vi "G2131-i仪器串口通讯.vi"(0 "VISA resource name":refnum<visa-resource-name>="COM3", 2 "baud rate (9600)":u32=9600) -> (1 "Delta2Min":string, 5 "H2O":string, 6 "12CO2":string, 7 "12CO2(dry）":string, 8 "Delta5Min":string, 9 "13CO2":string, 10 "13CO2（dry）":string)   [LabVIEW 2016]
uses:
  <vilib>/Instr/_visa.llb/VISA Configure Serial Port (Instr).vi
panel:
  out "返回数 2":u32
  out "read buffer":string
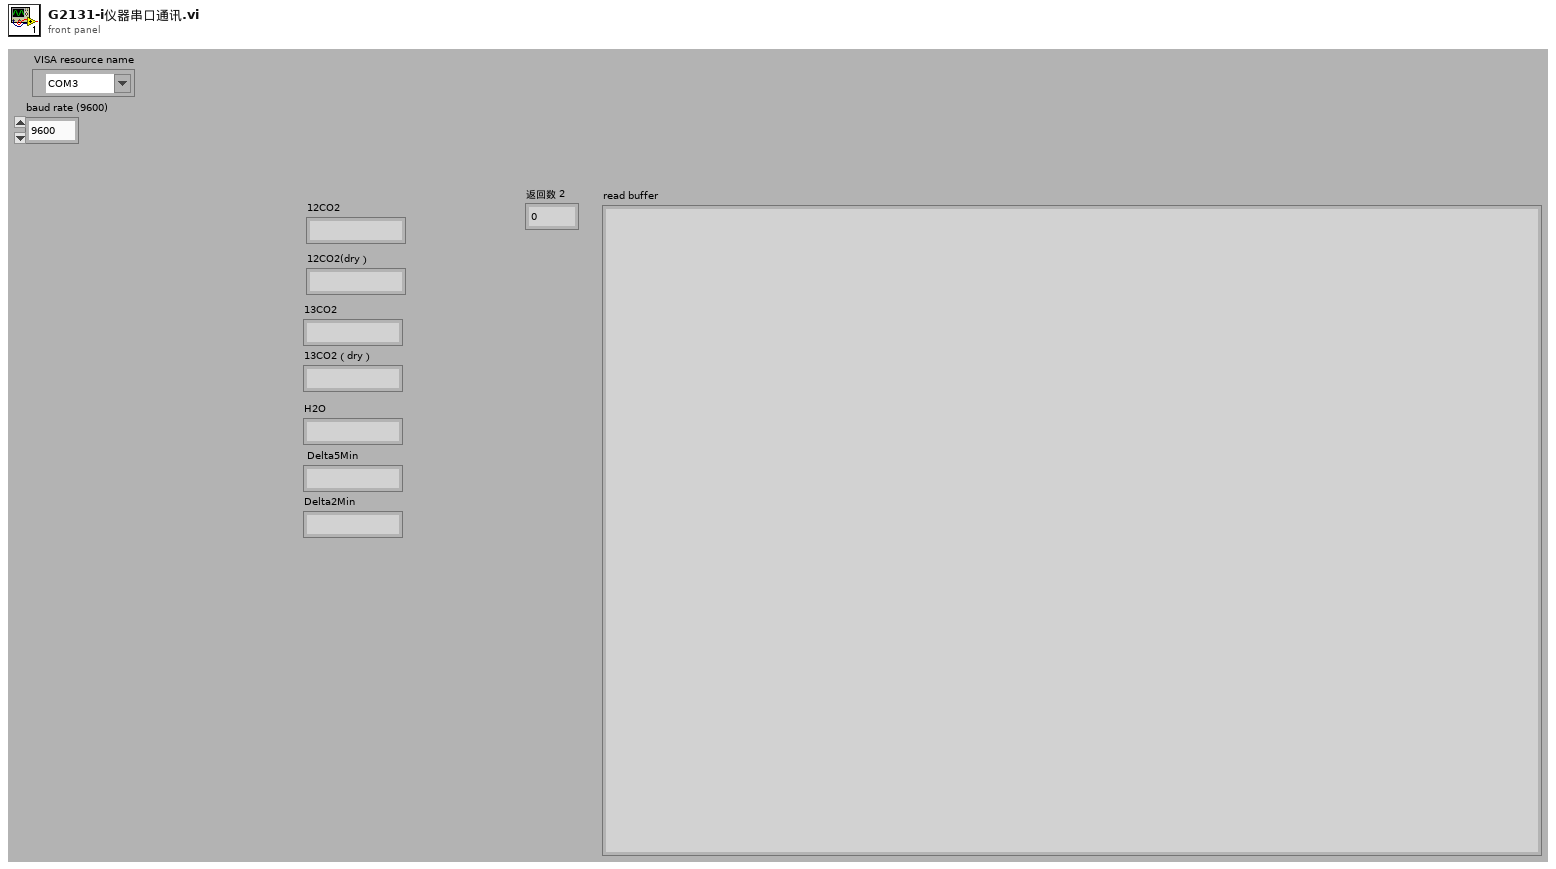
[diagram p1: front panel]
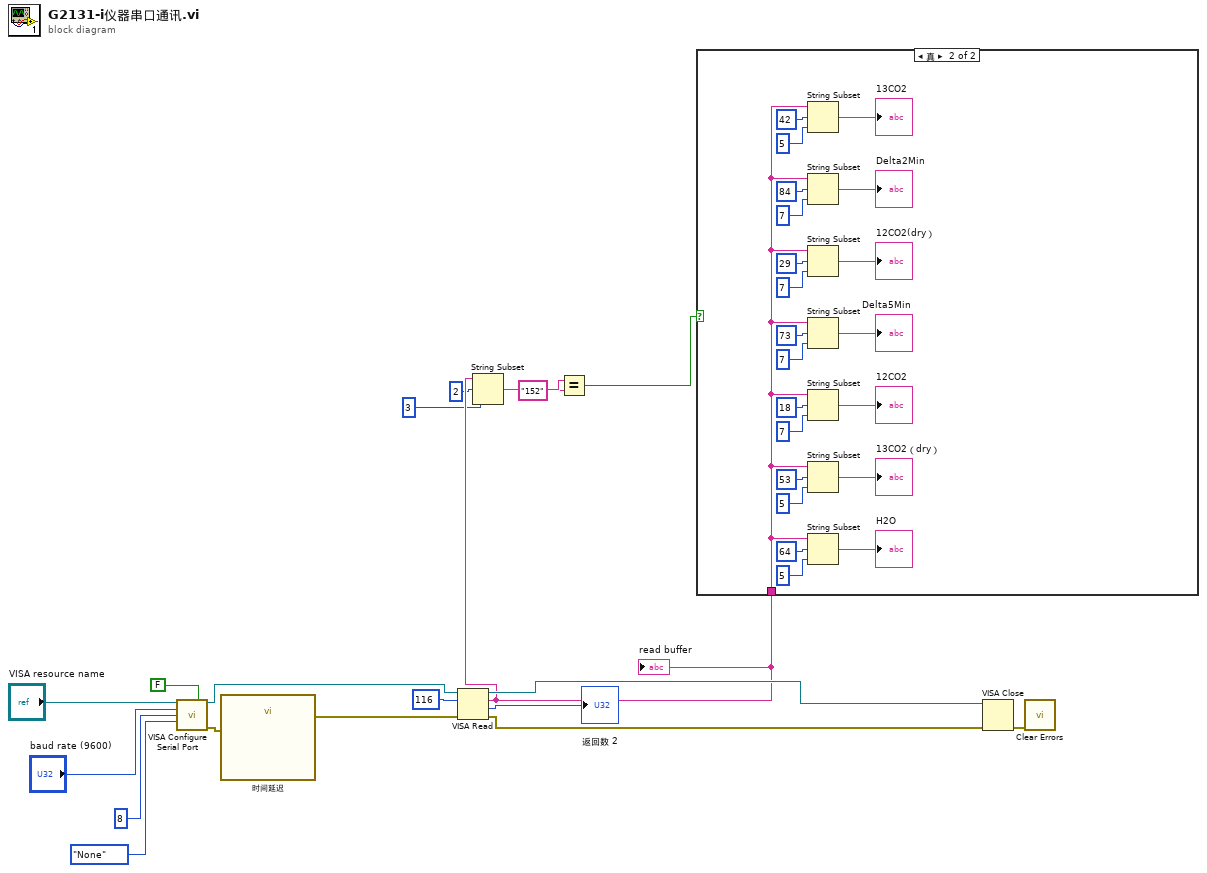
[diagram p0: block diagram]
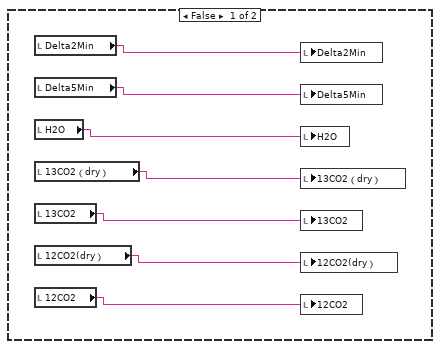
[diagram p2: hidden frame]
diagram:
  n1 = call-poly "VISA Configure Serial Port"("VISA resource name"="VISA resource name", "Enable Termination\nChar (T)"=FALSE ("Enable Termination\nChar (T)"), "baud rate (9600)"="baud rate (9600)", "data bits (8)"=u16 8, "parity (0:none)"=enum16{"None", "Odd", "Even", "Mark", "Space"}."None") -> ("VISA resource name out"=w9:refnum<visa-resource-name>, "error out"=w16:errorcluster)  [unwired: 9 in]
  n2 = call "时间延迟"("error in (no error)"=w16) -> ("error out"=w8:errorcluster)  [unwired: 10 in]
  n3 = VISA Read(VISA resource name=w9, byte count=u32 116 ("字节总数"), error in (no error)=w8) -> (VISA resource name out=w7:refnum<visa-resource-name>, read buffer=w6:string, return count=→"返回数 2":u32, error out=w15:errorcluster)
  "read buffer" <- w6
  n4 = String Subset(string=w6, offset (0)=2 ("偏移量(0)"), length (rest)=3 ("长度（剩余）")) -> (substring=w2:string)
  n5 = Equal?(x=w2, y="152") -> (x = y?=w3:bool)
  n6 = case shown="真" w3 {
    tunnel: w6 -> [_ w48]
    frame False {
      n7 = local read "Delta2Min"() -> (w20:string)
      n8 = local read "Delta5Min"() -> (w21:string)
      n9 = local read "H2O"() -> (w22:string)
      n10 = local read "13CO2（dry）"() -> (w23:string)
      n11 = local read "13CO2"() -> (w24:string)
      n12 = local read "12CO2(dry）"() -> (w25:string)
      n13 = local read "12CO2"() -> (w26:string)
      n14 = local write "Delta2Min"(w20) -> ()
      n15 = local write "Delta5Min"(w21) -> ()
      n16 = local write "H2O"(w22) -> ()
      n17 = local write "13CO2（dry）"(w23) -> ()
      n18 = local write "13CO2"(w24) -> ()
      n19 = local write "12CO2(dry）"(w25) -> ()
      n20 = local write "12CO2"(w26) -> ()
    }
    frame True {
      n21 = String Subset(string=w48, offset (0)=42 ("偏移量(0)"), length (rest)=5 ("长度（剩余）")) -> (substring=→"13CO2":string)
      n22 = String Subset(string=w48, offset (0)=84 ("偏移量(0)"), length (rest)=7 ("长度（剩余）")) -> (substring=→"Delta2Min":string)
      n23 = String Subset(string=w48, offset (0)=29 ("偏移量(0)"), length (rest)=7 ("长度（剩余）")) -> (substring=→"12CO2(dry）":string)
      n24 = String Subset(string=w48, offset (0)=73 ("偏移量(0)"), length (rest)=7 ("长度（剩余）")) -> (substring=→"Delta5Min":string)
      n25 = String Subset(string=w48, offset (0)=18 ("偏移量(0)"), length (rest)=7 ("长度（剩余）")) -> (substring=→"12CO2":string)
      n26 = String Subset(string=w48, offset (0)=53 ("偏移量(0)"), length (rest)=5 ("长度（剩余）")) -> (substring=→"13CO2（dry）":string)
      n27 = String Subset(string=w48, offset (0)=64 ("偏移量(0)"), length (rest)=5 ("长度（剩余）")) -> (substring=→"H2O":string)
    }
  }
  n28 = VISA Close(VISA resource name=w7, error in (no error)=w15) -> (error out=w12:errorcluster)
  n29 = call <vilib>:"Clear Errors.vi"("error in (no error)"=w12) -> ()  [unwired: 5 in, 2 out]
